vi "Con_Str_wDel.vi"(2 "Delimiter":string, 3 "Stringarray":string[](array[string])) -> (1 "Output":string)   [LabVIEW 2009]
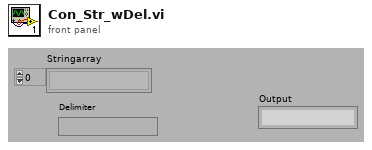
[diagram p1: front panel]
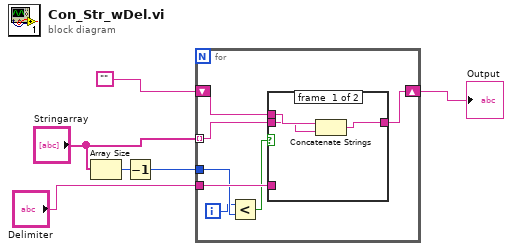
[diagram p0: block diagram]
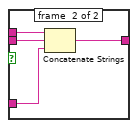
[diagram p2: hidden frame]
diagram:
  n1 = Array Size(array="Stringarray") -> (size(s)=w3:i32)
  n2 = Decrement(x=w3) -> (x-1=w1:i32)
  n3 = for {
    tunnel: "Stringarray" -> [w13] mode=indexing
    tunnel: "Delimiter" -> [w11]
    shift-right: [w10] -> w2
    shift-left: "" -> [w12]
    tunnel: w1 -> [w9]
    i -> [w8]
    n4 = Less?(x=w8, y=w9) -> (x < y?=w7:bool)
    n5 = case shown="False" w7 {
      tunnel: w13 -> [w15 w20]
      tunnel: w12 -> [w16 w19]
      tunnel: w11 -> [_ w18]
      tunnel: [w14 w17] -> w10
      frame #0 {
        n6 = Concatenate Strings(w16, w15) -> (w14:string)
      }
      frame #1 {
        n7 = Concatenate Strings(w19, w20, w18) -> (w17:string)
      }
    }
  }
  "Output" <- w2
